vi "Initialize TCP Send Resource.vi"(8 "error in (no error)":errorcluster, 11 "UR5 Robot in":refnum<class "UR5 Robot.lvclass">) -> (0 "error out":errorcluster, 3 "UR5 Robot out":refnum<class "UR5 Robot.lvclass">)   [LabVIEW 2018, in "UR5 Robot.lvlib" / "UR5 Robot.lvclass"]
uses:
  UR5 Robot.lvclass
  UR5 Robot.lvclass/UR5 Robot.ctl
  PPLs/Robot/Parent/Robot.lvlibp/Robot.lvclass
  C:/AME Test Engineering/LabVIEW/PPLs/Robot/Parent/Robot.lvlibp/Robot.lvclass
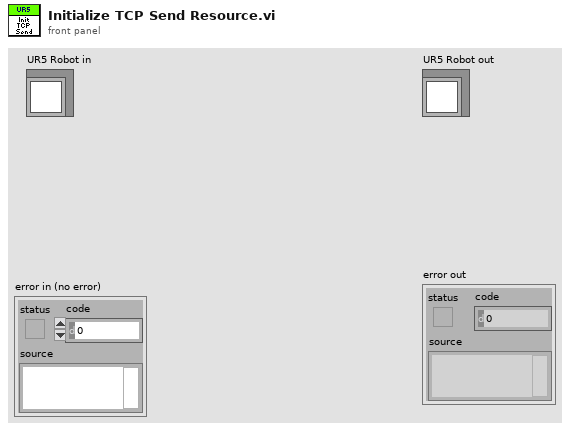
[diagram p1: front panel]
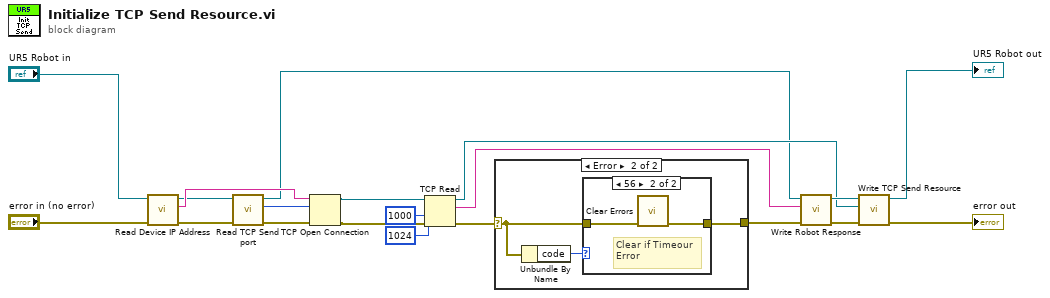
[diagram p0: block diagram]
diagram:
  n1 = call "Read Device IP Address.vi"("error in (no error)"="error in (no error)", "Robot in"="UR5 Robot in") -> ("error out"=w15:errorcluster, "Device IP Address"=w16:string, "Robot out"=w14:refnum<class "UR5 Robot.lvclass">)  [unwired: 7 in]
  n2 = call "Read TCP Send port.vi"("error in (no error)"=w15, "Robot in"=w14) -> ("error out"=w12:errorcluster, "TCP Send port"=w13:u16, "Robot out"=w1:refnum<class "UR5 Robot.lvclass">)  [unwired: 7 in]
  n3 = TCP Open Connection(address=w16, remote port or service name=w13, error in (no error)=w12) -> (connection ID=w3:refnum<k5>, error out=w4:errorcluster)  [unwired: 2 in]
  n4 = TCP Read(connection ID=w3, bytes to read=1024, error in (no error)=w4, 9:1000 ("timeout ms (25000)")) -> (connection ID out=w2:refnum<k5>, data out=w11:string, error out=w7:errorcluster)  [unwired: 1 in]
  n5 = case shown="Error" w7 {
    selector: w7 -> [w21 w23]
    tunnel: [w21 w22] -> w10
    frame No Error {
    }
    frame Error {
      n6 = Unbundle By Name(w23) -> ("code"=w24:i32)
      n7 = case shown="56" w24 {
        tunnel: w23 -> [w25 w27]
        tunnel: [w25 w26] -> w22
        frame 0, Default {
        }
        frame 56 {
          # "Clear if Timeour\nError"
          n8 = call <vilib>:"Clear Errors.vi"("error in (no error)"=w27) -> ("error out"=w26:errorcluster)  [unwired: 5 in, 1 out]
        }
      }
    }
  }
  n9 = call "Write Robot Response.vi"("error in (no error)"=w10, "Robot Response"=w11, "UR5 Robot in"=w1) -> ("error out"=w5:errorcluster, "UR5 Robot out"=w6:refnum<class "UR5 Robot.lvclass">)  [unwired: 7 in]
  n10 = call "Write TCP Send Resource.vi"("error in (no error)"=w5, "TCP Send Resource"=w2, "UR5 Robot in"=w6) -> ("error out"=→"error out":errorcluster, "UR5 Robot out"=→"UR5 Robot out":refnum<class "UR5 Robot.lvclass">)  [unwired: 7 in]
